vi "Insight_OPC.vi"(8 "error in (no error)":errorcluster, 11 "telnet connection":T1) -> (0 "error out":errorcluster, 1 "response data":string, 2 "OPC Bit value (1=Idle)":u32, 3 "telnet  connection out":T1)   [LabVIEW 2015]
doc: "Insight Photonic Solutions\n\nThis VI reads the operation complete (OPC) bit to determine if the laser has completed it's last requested action. For example, by polling the OPC bit through this VI the user can determine when sweep calibration has completed, before proceeding to the next task.\n\nThe OPC Bit is 1 when system is Idle, and 0 when system is Busy.\n\nver 1.0 - original release\nver 1.1 - added response data buffer as an output"
uses:
  Telnet Session.ctl
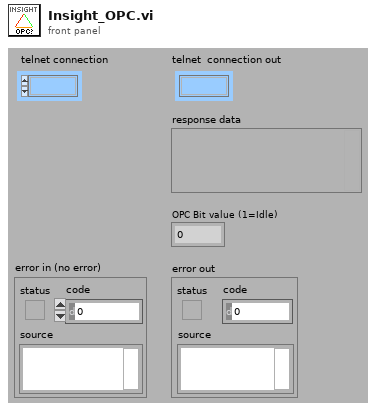
[diagram p1: front panel]
types:
  T1 = typedef "Telnet Session.ctl" = refnum<k1>
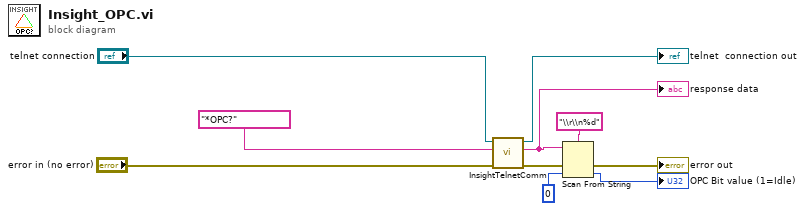
[diagram p0: block diagram]
diagram:
  n1 = call "InsightTelnetComm.vi"("error in"="error in (no error)", "write buffer (\"\")"="*OPC?" ("String"), "telnet connection"="telnet connection") -> ("error out"=w8:errorcluster, "response data"=w7:string, "telnet  connection out"=→"telnet  connection out":T1)  [unwired: 4 in]
  "response data" <- w7
  n2 = Scan From String(format string="\\r\\n%d", input string=w7, error in=w8, default 1=u32 0 ("default value 1")) -> (error out=→"error out":errorcluster, output 1=→"OPC Bit value (1=Idle)":u32)  [unwired: 1 in, 2 out]
